vi "user input.vi"(8 "error in":errorcluster, 11 "Interface":T1) -> (0 "error out":errorcluster, 3 "Inputs from system":T2)   [LabVIEW 2017, in "ThreePhasePLL runtime.lvclass"]
uses:
  ThreePhasePLL runtime.lvclass
  input user data.ctl
  <vilib>/NI/PowerElectronicsControl/ThreePhasePLL/Interface/InterfaceRef.ctl
  <instrlib>/_niInstr/Instruction Framework/v1/Host/Instruction Target/niInstr Instruction Target v1 Host.lvclass
  <instrlib>/_niInstr/Instruction Framework/v1/Host/Instruction Framework Context/niInstr Instruction Framework Context v1 Host.lvclass
  <vilib>/NI/PowerElectronicsControl/ThreePhasePLL/Interface/ThreePhasePLLInterface.lvlib
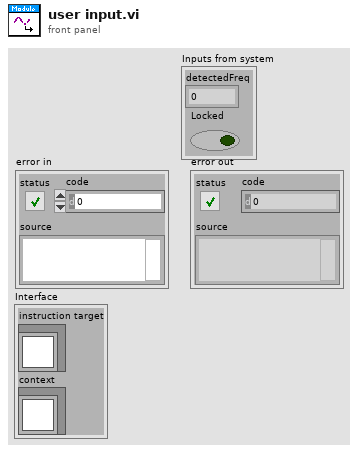
[diagram p1: front panel]
types:
  T1 = typedef "ThreePhasePLLInterface.lvlib/InterfaceRef.ctl" = cluster{"instruction target":refnum<class "niInstr Instruction Target v1 Host.lvclass">, "context":refnum<class "niInstr Instruction Framework Context v1 Host.lvclass">}
  T2 = typedef "ThreePhasePLL runtime.lvclass/input user data.ctl" = cluster{"detectedFreq":dbl, "Locked":bool}
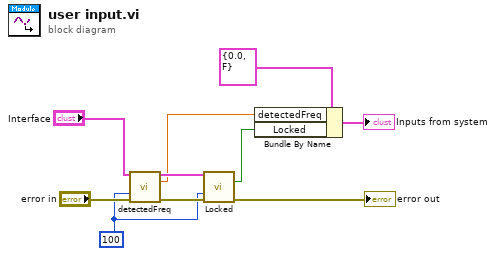
[diagram p0: block diagram]
diagram:
  w6 = 100 ("timeout (5000 ms)")
  n1 = call <vilib>:"detectedFreq.vi"("Interface in"="Interface", "timeout (5000 ms)"=w6, "error in"="error in") -> ("Interface out"=w8:T1, "detectedFreq"=w1:sgl, "error out"=w7:errorcluster)  [unwired: 10 in]
  n2 = call <vilib>:"Locked.vi"("Interface in"=w8, "timeout (5000 ms)"=w6, "error in"=w7) -> ("Locked"=w2:bool, "error out"=→"error out":errorcluster)  [unwired: 10 in, 1 out]
  n3 = Bundle By Name(cluster=T2 {"detectedFreq"=0.0, "Locked"=FALSE} ("Inputs from system"), "detectedFreq"=w1, "Locked"=w2) -> (→"Inputs from system":T2)
